vi "SP Create Plot Object.vi"(4 "Placement":T10, 6 "PlotChannel":T9={"ChIndex"=0, "Sxx"="", "Format"="", "Autoscale"=FALSE, "Scale"=0.0, "RefValue"=0.0, "RefPos"=0.0, "Fstart"=-1.0, "Fstop"=-1.0, "Funit"=enum."MHz", "Color"=enum."black", "DataQuery"="", "Markers"=FALSE}, 7 "Query":T1, 8 "error in (no error)":errorcluster, 9 "Name":string, 10 "Object Hierarchy (empty)":string[](array[string]), 11 "tdms file Ref":refnum<k34>) -> (0 "error out":errorcluster, 2 "new Object Hierarchy":string[](array[string]), 3 "dup tdms file Ref":refnum<k34>)   [LabVIEW 2011]
uses:
  server/dd/lib/Report Templates/Template TDM/enumObjectTypes.ctl
  server/dd/lib/Report Templates/Template TDM/objPlacement.ctl
  server/dd/lib/Report Templates/Template TDM/enumQueryResultTypes.ctl
  server/dd/lib/Report Templates/Template TDM/enumConditionType.ctl
  server/dd/lib/Report Templates/Template TDM/enumConditionOperator.ctl
  server/dd/lib/Report Templates/Template TDM/objQuery.ctl
  server/dd/lib/Report Templates/Template TDM/enumQueryKeyClass.ctl
  TypeDefs/SP Frequency Units.ctl
  server/dd/lib/Report Templates/Template TDM/enumColor.ctl
  server/dd/lib/Report Templates/Template TDM/enumSummaryOperator.ctl
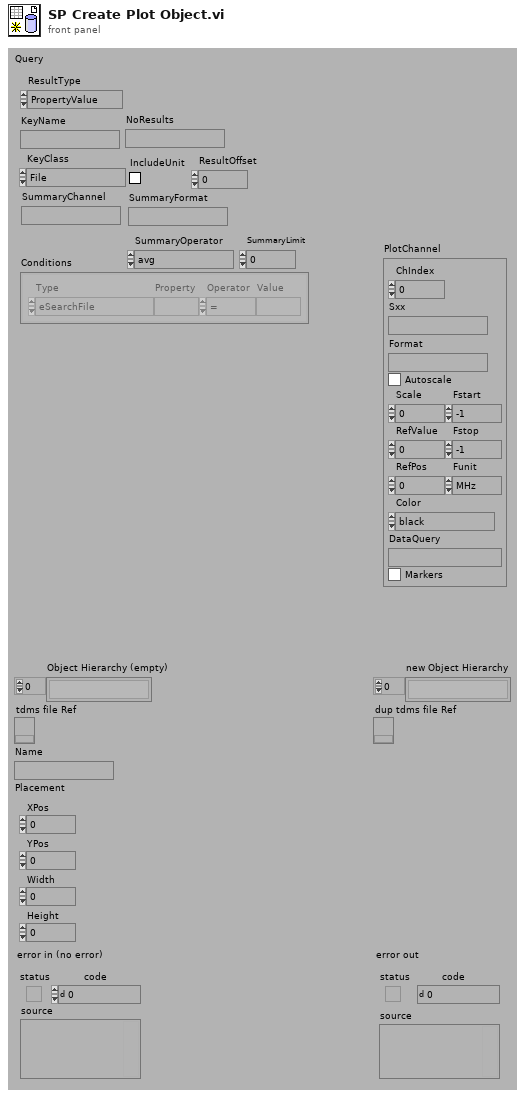
[diagram p1: front panel]
types:
  T1 = typedef "objQuery.ctl" = cluster{"ResultType":T2, "KeyName":string, "KeyClass":T3, "NoResults":string, "IncludeUnit":bool, "ResultOffset":i32, "SummaryChannel":string, "SummaryFormat":string, "SummaryOperator":T4, "SummaryLimit":i32, "Conditions":cluster{"Type":T5, "Property":string, "Operator":T6, "Value":string}[]}
  T2 = typedef "enumQueryResultTypes.ctl" = enum16{"PropertyValue", "Scalar", "Vector", "Summary"}
  T3 = typedef "enumQueryKeyClass.ctl" = enum16{"File", "Run", "Channel"}
  T4 = typedef "enumSummaryOperator.ctl" = enum16{"avg", "min", "max", "rng", "sum"}
  T5 = typedef "enumConditionType.ctl" = enum16{"eSearchFile", "eSearchChannelGroup", "eSearchChannel"}
  T6 = typedef "enumConditionOperator.ctl" = enum16{"="}
  T7 = typedef "SP Frequency Units.ctl" = enum16{"Hz", "kHz", "MHz", "GHz", "Points"}
  T8 = typedef "enumColor.ctl" = enum16{"black", "red", "green", "blue", "violet", "turquoise", "grey", "yell", "dark red", "dark green", "dark blue", "dark violet", "dark turquoise", "dark grey", "dark yellow", "white", "other colors", "no color"}
  T9 = cluster{"ChIndex":i32, "Sxx":string, "Format":string, "Autoscale":bool, "Scale":dbl, "RefValue":dbl, "RefPos":dbl, "Fstart":dbl, "Fstop":dbl, "Funit":T7, "Color":T8, "DataQuery":string, "Markers":bool}
  T10 = typedef "objPlacement.ctl" = cluster{"XPos":dbl, "YPos":dbl, "Width":dbl, "Height":dbl}
  T11 = typedef "enumObjectTypes.ctl" = enum16{"container", "graphics", "text", "picture", "qobject", "sparameterplot", "sparametertrace"}
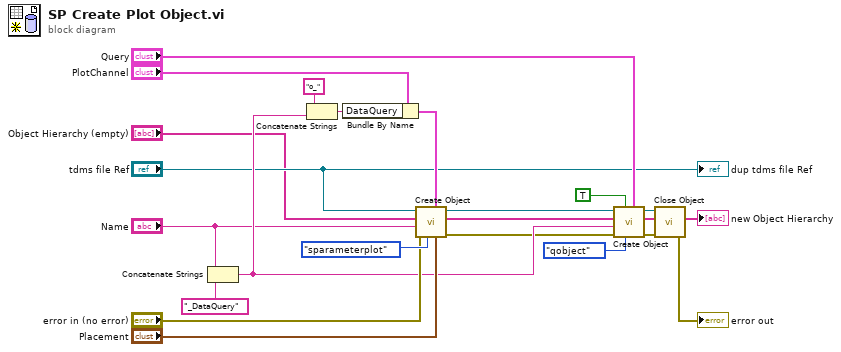
[diagram p0: block diagram]
diagram:
  n1 = Concatenate Strings("Name", "_DataQuery" ("Object Name")) -> (w17:string)
  n2 = Concatenate Strings("o_" ("Object Name"), w17) -> (w18:string)
  n3 = Bundle By Name(cluster="PlotChannel", "DataQuery"=w18) -> (w14:T9)
  n4 = call "Create Object.vi"("Object Placement"="Placement", "Properties"=w14, "Object Type (container)"=enumObjectTypes."sparameterplot", "error in (no error)"="error in (no error)", "Object Name (\"\")"="Name", "Object Hierarchy (empty)"="Object Hierarchy (empty)", "tdms file Ref"="tdms file Ref") -> ("error out"=w13:errorcluster, "new Object Hierarchy"=w6:string[], "dup tdms file Ref"=w10:refnum<k34>)  [unwired: 1 in, 1 out]
  n5 = call "Create Object.vi"("Properties"="Query", "Object Type (container)"=enumObjectTypes."qobject", "Supress Child Ref? (f)"=TRUE, "error in (no error)"=w13, "Object Name (\"\")"=w17, "Object Hierarchy (empty)"=w6, "tdms file Ref"=w10) -> ("error out"=w2:errorcluster, "new Object Hierarchy"=w5:string[], "dup tdms file Ref"=w1:refnum<k34>)  [unwired: 1 in, 1 out]
  n6 = call "Close Object.vi"("error in (no error)"=w2, "Object Hierarchy (empty)"=w5, "tdms file Ref"=w1) -> ("error out"=→"error out":errorcluster, "new Object Hierarchy"=→"new Object Hierarchy":string[])  [unwired: 3 out]
  "dup tdms file Ref" <- "tdms file Ref"
